vi "Quick Load Audio File (Path).vi"(8 "error in (no error)":errorcluster, 11 "Path":path) -> (0 "error out":errorcluster, 1 "data":waveform(i16)[](array[waveform]), 2 "Sample Rate":u32, 3 "Channels":u32, 4 "Codec":T1, 5 "PCM Frame Length":u64)   [LabVIEW 2020, in "G-Audio.lvlib"]
doc: "A single VI method to load an entire audio file from disk. The audio data will be returned as an I16 waveform array.\n\nNote this method is faster than reading audio chunks in a loop, but can result in higher peak memory allocation. If the file is very large, LabVIEW may run out of memory.\n\nSupported codecs: flac, mp3, ogg (vorbis), and wav."
uses:
  G-Audio.lvlib
  Controls/Audio File Codec.ctl
  Private/Result To Error.vi
  <vilib>/Utility/error.llb/Error Cluster From Error Code.vi
  Private/Copy Data.vi
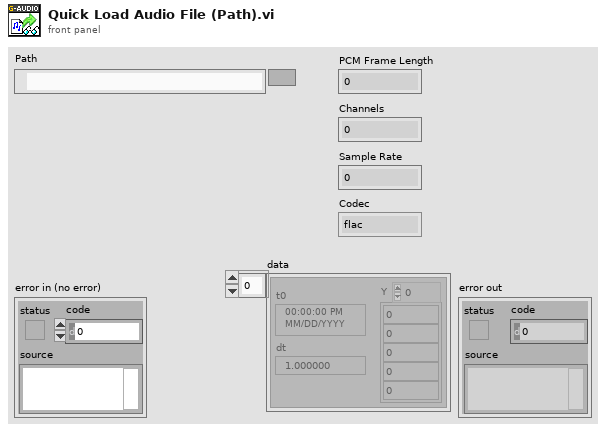
[diagram p1: front panel]
types:
  T1 = typedef "G-Audio.lvlib/Audio File Codec.ctl" = enum16{"flac", "mp3", "vorbis", "wav", "unsupported"}
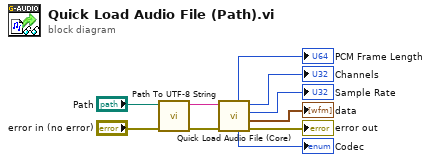
[diagram p0: block diagram]
diagram:
  n1 = call "Path To UTF-8 String.vi"("error in"="error in (no error)", "Path"="Path") -> ("error out"=w7:errorcluster, "UTF-8 String"=w9:string)  [unwired: 8 in]
  n2 = call "Quick Load Audio File (Core).vi"("error in (no error)"=w7, "Path"=w9) -> ("error out"=→"error out":errorcluster, "data"=→"data":waveform(i16)[], "Sample Rate"=→"Sample Rate":u32, "Channels"=→"Channels":u32, "Codec"=→"Codec":T1, "PCM Frame Length"=→"PCM Frame Length":u64)  [unwired: 4 in]
